vi "Parse I2C Messages.vi"(7 "Timestamp ID":T1, 8 "error in (no error)":errorcluster, 10 "User Timestamps":u64[](array[numeric])) -> (0 "error out":errorcluster, 2 "I2C Messages":string[][](array[string]), 3 "Count":i32)   [LabVIEW 2025]
uses:
  <instrlib>/FlexRIO/CSI-2/v2/FPGA/Types/Timestamp ID.ctl
  <instrlib>/FlexRIO/CSI-2/v2/FPGA/Types/Raw Timestamp.ctl
  <instrlib>/FlexRIO/CSI-2/v2/Host/subVIs/Convert Raw Timestamp to User Timestamp.vi
  <instrlib>/FlexRIO/CSI-2/v2/FPGA/NI CSI-2 API FPGA v2.lvlib
  <instrlib>/FlexRIO/CSI-2/v2/Host/NI CSI-2 API Host v2.lvlib
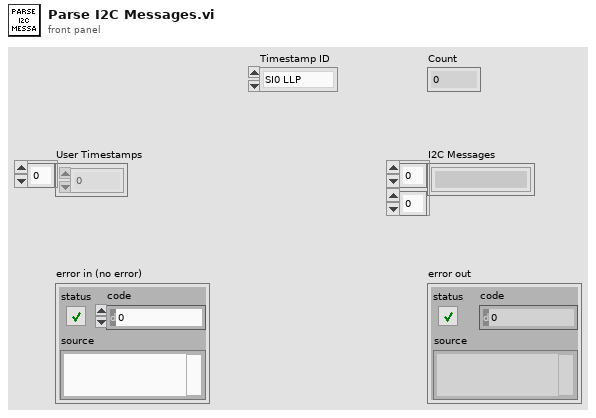
[diagram p1: front panel]
types:
  T1 = typedef "NI CSI-2 API FPGA v2.lvlib/Timestamp ID.ctl" = enum8{"SI0 LLP", "SI1 LLP", "SI2 LLP", "SI3 LLP", "SI4 LLP", "SI5 LLP", "SI6 LLP", "SI7 LLP", "SO0 LLP", "SO1 LLP", "SO2 LLP", "SO3 LLP", "SO4 LLP", "SO5 LLP", "SO6 LLP", "SO7 LLP", "Ser0 GPIO Bank", "Ser1 GPIO Bank", "Ser2 GPIO Bank", "Ser3 GPIO Bank", "Ser4 GPIO Bank", "Ser5 GPIO Bank", "Ser6 GPIO Bank", "Ser7 GPIO Bank", "Des0 GPIO Bank", "Des1 GPIO Bank", "Des2 GPIO Bank", "Des3 GPIO Bank", "Des4 GPIO Bank", "Des5 GPIO Bank", "Des6 GPIO Bank", "Des7 GPIO Bank", "User0", "User1", "User2", "User3", "User4", "User5", "User6", "User7", "User8", "User9", "User10", "User11", "User12", "User13", "User14", "User15", "User16", "User17", "User18", "User19", "User20", "User21", "User22", "User23", "User24", "User25", "User26", "User27", "User28", "User29", "User30", "User31"}
  T2 = typedef "NI CSI-2 API FPGA v2.lvlib/Raw Timestamp.ctl" = cluster{"timestamp":u64, "valid":bool}
  T3 = typedef "NI CSI-2 API FPGA v2.lvlib/User Timestamp.ctl" = cluster{"valid":bool, "user data":fxp<+,58,58>, "id":T1}
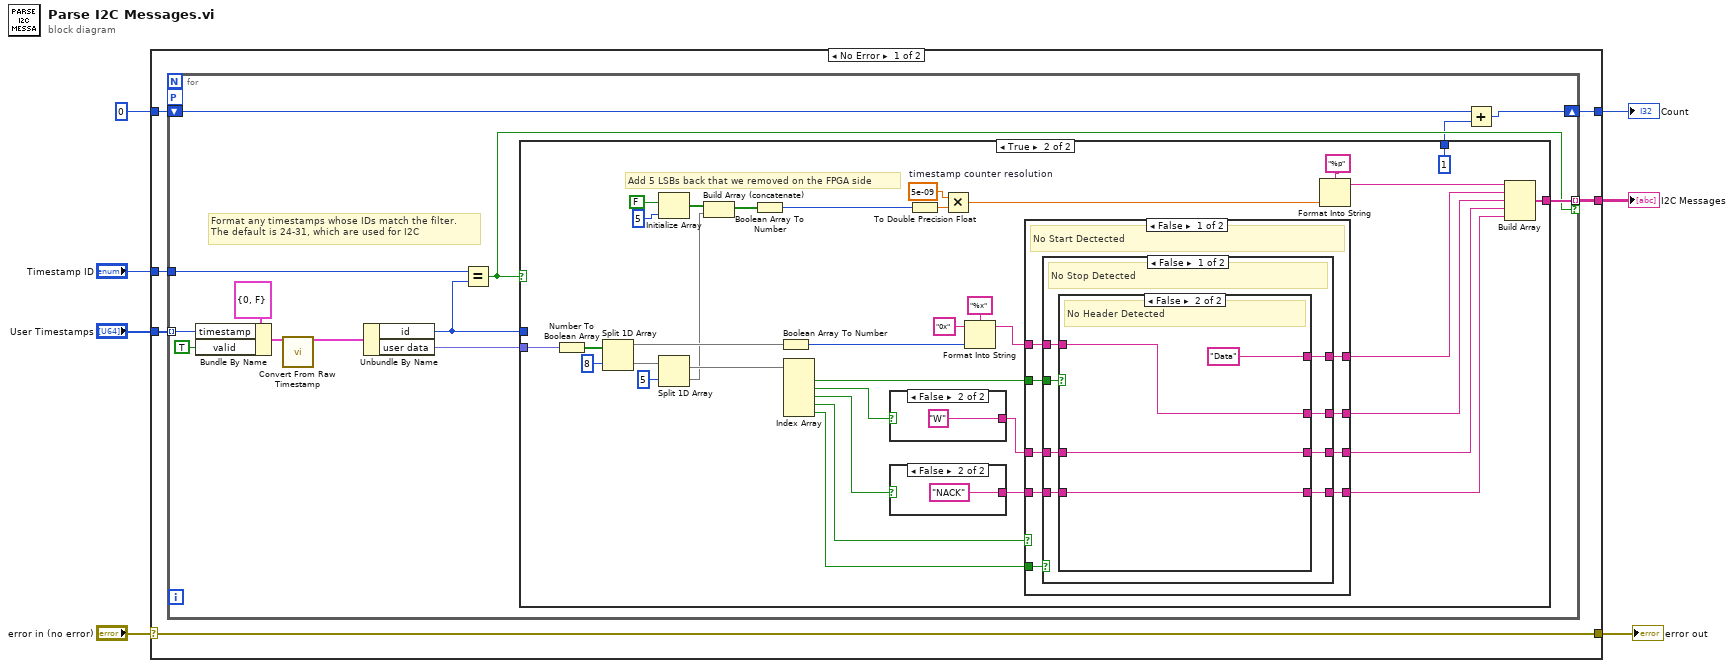
[diagram p0: block diagram]
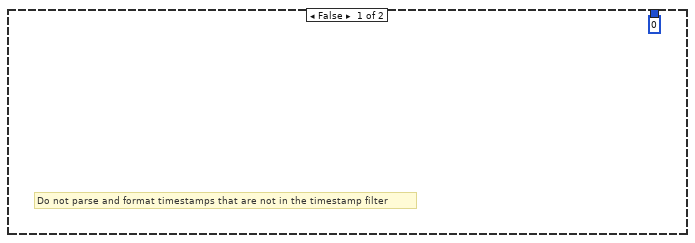
[diagram p2: hidden frame]
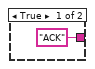
[diagram p3: hidden frame]
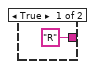
[diagram p4: hidden frame]
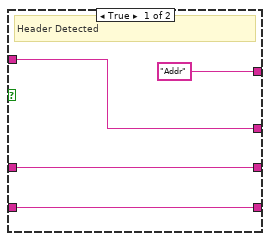
[diagram p5: hidden frame]
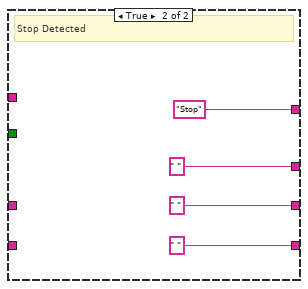
[diagram p6: hidden frame]
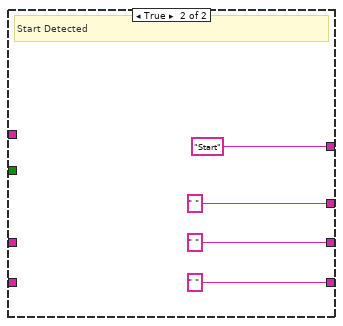
[diagram p7: hidden frame]
diagram:
  n1 = case shown="No Error" "error in (no error)" {
    selector: "error in (no error)" -> [w8 w100]
    tunnel: "User Timestamps" -> [w13 _]
    tunnel: "Timestamp ID" -> [w12 _]
    tunnel: 0 -> [w11 _]
    tunnel: [w10 _] -> w4
    tunnel: [w9 _] -> w3
    tunnel: [w8 w100] -> w1
    frame No Error {
      n2 = for {
        tunnel: [w26] -> w10 mode=indexing if=w23
        workers-P: _ -> [_]
        shift-right: [w21] -> w9
        shift-left: w11 -> [w20]
        tunnel: w12 -> [w19]
        tunnel: w13 -> [w15] mode=indexing
        # "Format any timestamps whose IDs match the filter.\nThe default is 24-31, which are used for I2C"
        n3 = Bundle By Name(cluster=T2 {"timestamp"=0, "valid"=FALSE} ("raw timestamp"), "timestamp"=w15, "valid"=TRUE) -> (w17:T2)
        n4 = call-poly <instrlib>:"Convert From Raw Timestamp.vi"("raw timestamp"=w17) -> ("user timestamp"=w14:T3)  [unwired: 14 in]
        n5 = Unbundle By Name(w14) -> ("id"=w24:T1, "user data"=w25:fxp<+,58,58>)
        n6 = Equal?(x=w19, y=w24) -> (x = y?=w23:bool)
        n7 = case shown="True" w23 {
          tunnel: [_ w61] -> w26
          tunnel: w25 -> [_ w56]
          tunnel: w24 -> [_ _]
          tunnel: [0 ("x") 1 ("x")] -> w22
          frame False {
            # "Do not parse and format timestamps that are not in the timestamp filter"
          }
          frame True {
            w59 = 5e-09  # timestamp counter resolution
            # "Add 5 LSBs back that we removed on the FPGA side"
            n8 = Number To Boolean Array(number=w56) -> (Boolean array=w55:bool[])
            n9 = Split 1D Array(array=w55, index=8) -> (first subarray=w50:bool[], second subarray=w53:bool[])
            n10 = Initialize Array(FALSE, 5 ("dimension size")) -> (w47:bool[])
            n11 = Split 1D Array(array=w53, index=5) -> (first subarray=w51:bool[], second subarray=w46:bool[])
            n12 = Build Array (concatenate)(w47, w46) -> (w45:bool[])
            n13 = Boolean Array To Number(Boolean array=w45) -> (number=w44:u64)
            n14 = Boolean Array To Number(Boolean array=w50) -> (number=w31:u32)
            n15 = Index Array(array=w51) -> (element #1=w41:bool, element #2=w40:bool, element #3=w37:bool, element #4=w43:bool, element #5=w42:bool)  [unwired: 5 in]
            n16 = case shown="False" w40 {
              tunnel: ["R" "W"] -> w39
              frame True {
              }
              frame False {
              }
            }
            n17 = case shown="False" w37 {
              tunnel: ["ACK" "NACK"] -> w38
              frame True {
              }
              frame False {
              }
            }
            n18 = To Double Precision Float(number=w44) -> (double precision float=w58:dbl)
            n19 = Multiply(x=w59, y=w58) -> (x*y=w60:dbl)
            n20 = Format Into String(format string="%x", initial string="0x", w31) -> (resulting string=w30:string)  [unwired: 1 in, 1 out]
            n21 = case shown="False" w43 {
              tunnel: w42 -> [w75 _]
              tunnel: w41 -> [w74 _]
              tunnel: w39 -> [w73 _]
              tunnel: w38 -> [w72 _]
              tunnel: w30 -> [w71 _]
              tunnel: [w70 "Start"] -> w36
              tunnel: [w69 " "] -> w29
              tunnel: [w68 " "] -> w35
              tunnel: [w67 " "] -> w34
              frame False {
                # "No Start Dectected"
                n22 = case shown="False" w75 {
                  tunnel: w74 -> [w83 _]
                  tunnel: w73 -> [w82 _]
                  tunnel: w72 -> [w81 _]
                  tunnel: w71 -> [w80 _]
                  tunnel: [w79 "Stop"] -> w70
                  tunnel: [w78 " "] -> w69
                  tunnel: [w77 " "] -> w68
                  tunnel: [w76 " "] -> w67
                  frame False {
                    # "No Stop Detected"
                    n23 = case shown="False" w83 {
                      tunnel: w82 -> [w85 w89]
                      tunnel: w81 -> [w84 w88]
                      tunnel: w80 -> [w86 w90]
                      tunnel: ["Addr" "Data"] -> w79
                      tunnel: [w86 w90] -> w78
                      tunnel: [w85 w89] -> w77
                      tunnel: [w84 w88] -> w76
                      frame True {
                        # "Header Detected"
                      }
                      frame False {
                        # "No Header Detected"
                      }
                    }
                  }
                  frame True {
                    # "Stop Detected"
                  }
                }
              }
              frame True {
                # "Start Detected"
              }
            }
            n24 = Format Into String(format string="%p", w60) -> (resulting string=w62:string)  [unwired: 2 in, 1 out]
            n25 = Build Array(w62, w36, w29, w35, w34) -> (w61:string[])
          }
        }
        n26 = Add(x=w20, y=w22) -> (x+y=w21:i32)
      }
    }
    frame Error {
    }
  }
  "I2C Messages" <- w4
  "Count" <- w3
  "error out" <- w1
